vi "check source version AC.vi"() -> (0 "continue running?":bool, 1 "Newer version available":bool, 2 "year":i32, 3 "application name":string, 4 "Application folder":path, 6 "error out":errorcluster)   [LabVIEW 2010]
uses:
  version state.ctl
  <vilib>/Platform/browser.llb/Open URL in Default Browser (string).vi
panel:
  out "data":string
  out "version state":T1
  out "this version":path
  out "This version":timestamp
  out "time stamp":timestamp
  out "Connection":string
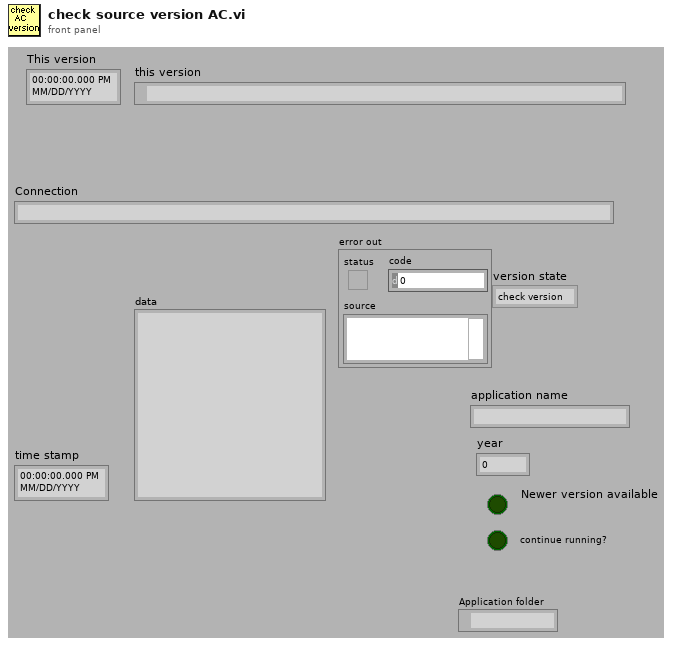
[diagram p1: front panel]
types:
  T1 = typedef "version state.ctl" = enum16{"check version", "prompt for update", "go to download", "accept license", "display copyright", "done"}
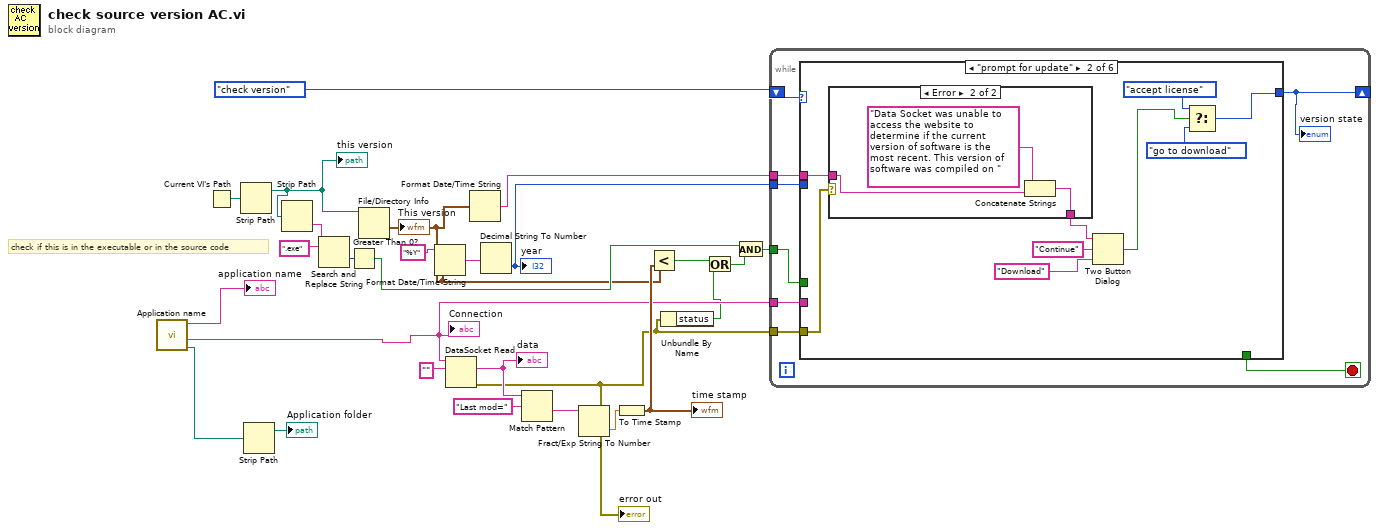
[diagram p0: block diagram]
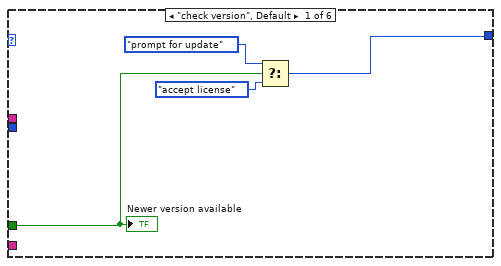
[diagram p2: hidden frame]
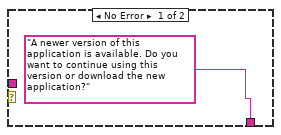
[diagram p3: hidden frame]
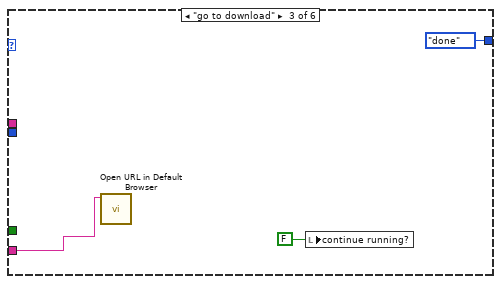
[diagram p4: hidden frame]
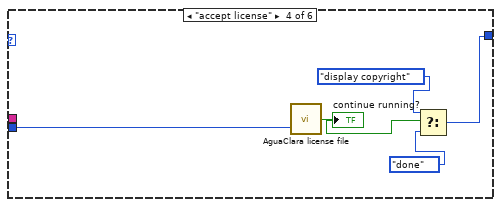
[diagram p5: hidden frame]
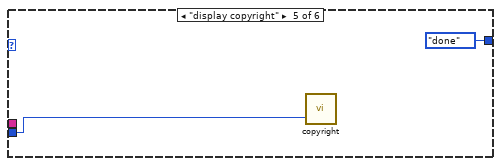
[diagram p6: hidden frame]
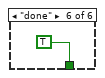
[diagram p7: hidden frame]
diagram:
  # "check if this is in the executable or in the source code"
  n1 = call "Application name.vi"() -> ("Ini file path"=w9:path, "download site"=w10:string, "application name"=→"application name":string)  [unwired: 4 in, 1 out]
  "Connection" <- w10
  n2 = Current VI's Path() -> (path=w25:path)
  n3 = Strip Path(path=w25) -> (stripped path=w15:path)  [unwired: 1 out]
  "this version" <- w15
  n4 = Strip Path(path=w9) -> (stripped path=→"Application folder":path)  [unwired: 1 out]
  n5 = Strip Path(path=w15) -> (name=w16:string)  [unwired: 1 out]
  n6 = Search and Replace String(input string=w16, search string=".exe") -> (offset past replacement=w17:i32)  [unwired: 6 in, 3 out]
  n7 = Greater Than 0?(x=w17) -> (x > 0?=w14:bool)
  n8 = File/Directory Info(path=w15) -> (last mod=w2:timestamp)  [unwired: 1 in, 6 out]
  "This version" <- w2
  n9 = Format Date/Time String(time format string (%c)="%Y", seconds (now)=w2) -> (date/time string=w3:string)  [unwired: 1 in]
  n10 = DataSocket Read(10:"" ("text"), 11:w10) -> (0:w4:errorcluster, 2:w21:string)  [unwired: 3 in, 5 out]
  "data" <- w21
  "error out" <- w4
  n11 = Format Date/Time String(seconds (now)=w2) -> (date/time string=w1:string)  [unwired: 2 in]
  n12 = Decimal String To Number(string=w3) -> (number=w20:i32)  [unwired: 2 in, 1 out]
  "year" <- w20
  n13 = Match Pattern(string=w21, regular expression="Last mod=") -> (after substring=w23:string)  [unwired: 1 in, 3 out]
  n14 = Fract/Exp String To Number(string=w23) -> (number=w24:dbl)  [unwired: 3 in, 1 out]
  n15 = To Time Stamp(1:w24) -> (0:w26:timestamp)
  "time stamp" <- w26
  n16 = Less?(x=w2, y=w26) -> (x < y?=w7:bool)
  n17 = Unbundle By Name(w4) -> ("status"=w5:bool)
  n18 = Or(x=w7, y=w5) -> (x .or. y?=w6:bool)
  n19 = And(x=w14, y=w6) -> (x .and. y?=w13:bool)
  n20 = while {
    shift-right: [w35] -> _
    shift-left: version_state."check version" ("version state") -> [w34]
    tunnel: w13 -> [w33]
    tunnel: w10 -> [w32]
    tunnel: w20 -> [w31]
    tunnel: w4 -> [w29]
    tunnel: w1 -> [w28]
    stop <- w30 stop-if-true
    n21 = case shown="\"prompt for update\"" w34 {
      tunnel: [w39 w46 version_state."done" ("version state") w57 version_state."done" ("version state") _] -> w35
      tunnel: w33 -> [w36 _ _ _ _ _]
      tunnel: w32 -> [_ _ w53 _ _ _]
      tunnel: w31 -> [_ _ _ w60 w62 _]
      tunnel: [_ _ _ _ _ TRUE] -> w30
      tunnel: w29 -> [_ w45 _ _ _ _]
      tunnel: w28 -> [_ w40 _ _ _ _]
      frame "check version", Default {
        n22 = Select(t=version_state."prompt for update" ("version state"), s=w36, f=version_state."accept license" ("version state")) -> (s? t:f=w39:T1)
        "Newer version available" <- w36
      }
      frame "prompt for update" {
        n23 = case shown="Error" w45 {
          tunnel: ["A newer version of this application is available. Do you want to continue using this version or download the new application?" ("message") w50] -> w41
          tunnel: w40 -> [_ w52]
          frame No Error {
          }
          frame Error {
            n24 = Concatenate Strings("Data Socket was unable to access the website to determine if the current version of software is the most recent. This version of software was compiled on " ("message"), w52) -> (w50:string)
          }
        }
        n25 = Two Button Dialog(message=w41, 1:"Download" ("F button name (\"Cancel\")"), 2:"Continue" ("T button name (\"OK\")")) -> (T button?=w42:bool)
        n26 = Select(t=version_state."accept license" ("version state"), s=w42, f=version_state."go to download" ("version state")) -> (s? t:f=w46:T1)
      }
      frame "go to download" {
        n27 = call-poly <vilib>:"Open URL in Default Browser.vi"("URL"=w53) -> ()  [unwired: 5 in, 2 out]
        n28 = local write "continue running?"(FALSE ("continue running?")) -> ()
      }
      frame "accept license" {
        n29 = call "AguaClara license file.vi"("year"=w60) -> ("Accepted"=w59:bool)  [unwired: 1 in]
        "continue running?" <- w59
        n30 = Select(t=version_state."display copyright" ("version state"), s=w59, f=version_state."done" ("version state")) -> (s? t:f=w57:T1)
      }
      frame "display copyright" {
        n31 = call "copyright.vi"("year"=w62) -> ()  [unwired: 3 in]
      }
      frame "done" {
      }
    }
    "version state" <- w35
  }
